vi "AlliGator All ROIs Average Lifetimes.vi"(8 "error in (no error)":errorcluster, 10 "Lifetime Graph":refnum<vi>, 11 "AlliGator Internal Variables DVR":refnum<data-value>) -> (0 "error out":errorcluster, 1 "Message":string, 3 "AlliGator Internal Variables DVR":refnum<data-value>)   [LabVIEW 2021, in "AlliGator Decay Processing.lvlib"]
doc: "Computes an approximate average lifetime for all ROI decays, based on the integral under the curve and IRF information."
uses:
  AlliGator Decay Processing.lvlib
  Internal Variables/AlliGator Internal Variables v2.ctl
  <vilib>/vision/Image Controls.llb/IMAQ Image.ctl
  Internal Variables/AlliGator Gate Image Set.ctl
  Files/AlliGator FLI Dataset Type.ctl
  Files/AlliGator Data Series Type.ctl
  Dual-Channel Datasets/AlliGator Dataset Channel.ctl
  Settings/AlliGator Gate Arithmetic.ctl
  Source Image/AlliGator Displayed Image.ctl
  Image/Named ROI Description.ctl
  Phasor Graph/AlliGator Decay Metadata v3.ctl
  Decay Preprocessing/AlliGator Decay Background Subtraction Info.ctl
  Decay Preprocessing/AlliGator Baseline Subtraction Method.ctl
  Graphs/XY Graph/XY Graph Plot Shift Parameters.ctl
  Graphs/XY Graph/XY Graph Plot Shift Method.ctl
  Decay Preprocessing/AlliGator Decay Extrapolation Parameters.ctl
  Phasor/Calibration Phasor (m, phi).ctl
  Phasor/Phasor Reference Series.ctl
  Phasor/Phasor Calibration Map v2.ctl
  Phasor/Phasor (g, s).ctl
  Phasor Graph/AlliGator Raw Phasor Plot Data v5.ctl
  Phasor/Phasor Standard Deviation Options.ctl
  Phasor Plot/AlliGator Phasor Multi-Harmonic Data.ctl
  Phasor/Phasor Harmonic Data.ctl
  Decay Fit Parameter Map/AlliGator Decay Fit Options & Parameters v4.ctl
  Fits/Decay Convolution/Decay Model.ctl
  Fits/Residual Type.ctl
  Fits/Non-linear Fitting Method v2.ctl
  Fits/Fit Calculation Method.ctl
  Fits/Non-linear Fitting Algorithm.ctl
  Decay Preprocessing/AlliGator Decay Preprocessing Parameters.ctl
  Fits/IRF(X)PSED/Decay Fit Parameters & Derived Quantities List v2.ctl
  Fits/IRF(X)PSED/Decay Fit Result Constraint.ctl
  Decay Fit Parameter Map/AlliGator Parameter Maps Data.ctl
  Globals, Variables, Constants/AlliGator Variables List.ctl
  Settings/AlliGator Average Lifetime Options.ctl
  Settings/AlliGator Settings List.ctl
  Rich Text Box/Text Format List.ctl
  Variant/Variant to Data/Variant to U16.vi
  Variant/Variant to Data/Variant to Boolean.vi
  Globals, Variables, Constants/AlliGator Abort.vi
  <vilib>/Utility/error.llb/Error Cluster From Error Code.vi
  <vilib>/ErrorRing/Error Ring.xnode
  Fits/IRF(X)PSED/MLE Baseline Offset Type.ctl
  Decay Fit/AlliGator Decay Fit Parameter Constraints 2.ctl
  Fits/IRF(X)PSED/Decay Fit Parameters In List.ctl
  Globals, Variables, Constants/AlliGator Globals, Variables & Constants.lvlib
  Image/Image.lvlib
  Source Image/AlliGator Source Image.lvlib
  Strings/Strings.lvlib
  Time/Time.lvlib
  Graphs/XY Graph/XY Graph Add-Ons.lvlib
  Settings/AlliGator Settings.lvlib
  Decay Preprocessing/AlliGator Decay Preprocessing.lvlib
  Variant/Variant to Data/Variant to Data.lvlib
  Notebook/Notebook.lvlib
  Fits/Fits.lvlib
  IRF/AlliGator IRF.lvlib
  Utilities/Utilities.lvlib
  GUI/GUI.lvlib
  Decay Fit Parameter Map/AlliGator Decay Fit Parameter Map.lvlib
  Decay Fit/AlliGator Decay Fit.lvlib
  Fits/IRF(X)PSED/Fit Weights Type v2.ctl
  Fits/IRF(X)PSED/Decay Fit Options v4.ctl
  Phasor/Phasor.lvlib
  Files/AlliGator Files.lvlib
  Internal Variables/AlliGator Internal Variables.lvlib
  Phasor Graph/AlliGator Phasor Graph.lvlib
  Phasor Plot/AlliGator Phasor Plot.lvlib
  Dual-Channel Datasets/AlliGator Dual-Channel Datasets.lvlib
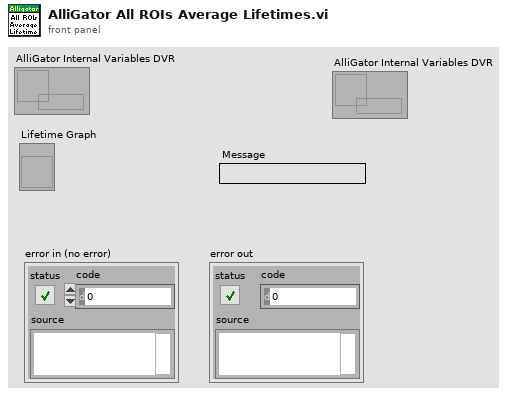
[diagram p1: front panel]
types:
  T1 = typedef "AlliGator Globals, Variables & Constants.lvlib/AlliGator Variables List.ctl" = enum16{"---- GUI ----", "GUI:Initialization Status", "GUI:State Indicators Refnum", "GUI:Original AlliGator Menu Items", "GUI:Current Action Loop State", "GUI:Script in progress", "GUI:Playback", "GUI:Loop Playback", "GUI:Search ROI Used", "GUI:Search ROI", "Decay Graph Max Legend Size", "Intensity Graph Max Legend Size", "Decay Statistics Graph Max Legend Size", "Phasor Graph Max Legend Size", "Phasor Ratio Graph Max Legend Size", "Lifetime Graph Max Legend Size", "---- Files ----", "Files:Export Dataset Frames as Individual Files", "Files:Show Batch Export Help Balloons", "Files:Frames in Dataset", "Files:ptu File Frame Start Indices", "Files:Current Frame in Dataset", "Files:Current Frame Timestamp", "Files:Dataset Loaded", "Files:Dataset Metadata", "Files:Dataset Channel", "Files:Dataset Data Description", "Files:Background Dataset Metadata", "Files:Background Dataset Channel", "Files:Background Dataset Data Description", "Files:Background File Subtraction", "Files:Background File Path", "Files:Background File Pile-up Correction", "Files:Background File Pixel Well Capacity", "Files:Background File Scaling Factor", "Files:Current Dataset Load Settings", "Files:Dataset Path", "Files:ICCD-specific Information", "Files:Macrotime Gate Separation", "------ Python Plugins ------", "Python Plugins:Information", "Python Plugins:Python Session", "Python Plugins:Valid Python Session?", "---- Source Image ----", "Source Image:ROIs", "Source Image:Current ROI", "Source Image:ROI Event Refnum", "X_Source Image:Display Range", "X_Source Image:Palette Information", "X_Source Image:Type of Displayed Image", "X_Time Gate Slider", "Source Image:Palette List", "Source Image:Scale", "Source Image:ROI Overlay Color", "Source Image:Overlay to Erase", "Source Image:Is Displayed Image Accumulated", "Source Image:White Light Image Modified", "Source Image:Mask Image Modified", "---- Image Profile Window ----", "Image Profile:Window Event Refnum", "Image Profile:IntensityType", "Image Profile:Intensity Average Type", "Image Profile:Intensity-weighted SDV", "Image Profile:Box Profile Type", "Image Profile:Window Open", "Image Profile:Plotted Fit Parameter", "------ Phasor Graph -------", "Phasor Graph:Show Line", "---- Phasor Plot ---", "Phasor Plot:Parameters Changed", "Phasor Plot:FLI Dataset Modified since last Calculation", "Phasor Harmonics Data", "Selected Phasor Harmonics", "Phasor Harmonic Manager Event Refnum", "Phasor Plot:ROIs", "Phasor Plot:Current ROI", "Phasor Plot:ROI Event Refnum", "Phasor Plot:Image Reference Points", "Phasor Plot:Computed", "Phasor Plot:Palette Information", "Phasor Plot:Palette List", "Phasor Plot:Phasor Ratio Palette Information", "Phasor Plot:Phasor Ratio Palette List", "Phasor Plot:Image Scale", "Phasor Plot:Image Overlay to Erase", "Phasor Plot:Image Elements to Update", "Phasor Plot:Current Calculation Parameters", "Phasor Plot:Current Calibration Options", "Phasor Plot:Reset Cumulated Phasor Plot", "Phasor Plot:Reference 1", "Phasor Plot:Lifetime Reference 1", "Phasor Plot:Reference 1 Frequency", "Phasor Plot:Reference 2", "Phasor Plot:Lifetime Reference 2", "Phasor Plot:Reference 2 Frequency", "---- Decay Analysis ----", "Number of Selected Decays to Fit", "LS Fit Results", "LAR Fit Results", "BS Fit Results", "Last Decay Max - Min", "Best Fit Parameters", "Best Fit Parameter Names", "Actual Size X", "Actual Size Y", "Binning X", "Binning Y", "Actual # Gates", "Dataset Number", "Gates to...", "Gates Skipped", "Gates to keep", "Gate Step", "Gate Separation", "Reversed Gates", "Pile-up Correction", "Pixel Well Capacity", "Background Subtracted", "Background Subtraction Method", "Background Definition Range", "Background File (deprecated)", "Number of Dataset Accumulated", "Array of Accumulated Dataset Paths", "Do Averaged Datasets", "Destination File Path", "Process Plot Target", "Use 1/D as Phasor Frequency", "---- Decay Fit Parameter Map -----", "Decay Fit Parameter Map:Palette Information", "Decay Fit Parameter Map:Palette List", "Decay Fit Parameter Map:X Resolution", "Decay Fit Parameter Map:Y Resolution", "Decay Fit Parameter Map:Use Decay Fit Result Constraints", "Decay Fit Parameter Map:Decay Fit Result Constraints", "Decay Fit Parameter Map:Decay Fit Result Constraints Applied", "---- Parameter Map ----", "Parameter Map:Palette Information", "Parameter Map:Palette List", "------- Local Decay Window ---------", "Local Decay Graph Window:Event Refnum", "Local Decay Graph Window:Use normalized IRF for convolution", "----- Miscellaneous ----", "Misc:Skippable Dialog Windows Status"}
  T2 = typedef "AlliGator Settings.lvlib/AlliGator Average Lifetime Options.ctl" = cluster{"Use Local IRF ":bool, "Use IRF Offset":bool, "Use Fixed Offset":bool, "Fixed Offset":dbl[unit], "Baseline %":dbl}
  T3 = typedef "AlliGator Settings.lvlib/AlliGator Settings List.ctl" = enum16{"GUI:Visible Settings Tab", "GUI:Last Run Version", "Source Image:Use Image Histogram for Contrast", "Source Image:Low Count Pixels Rejection Options", "Source Image:High Count Pixels Rejection Options", "Source Image:Use Image Brightness", "Source Image:Blend Overlay with Image Background", "Source Image:Use Fixed ROI Diameter", "Source Image:ROI Diameter", "Source Image:ROI Center Color", "Source Image:Peak Threshold", "Source Image:Intensity Threshold", "Source Image:Image Binning Options", "Source Image:Image Smoothing Options", "Source Image:Image Histogram Active", "Source Image:Invert Binary Mask", "Source Image:Hot Pixel Removal", "Source Image:Overlay Analyzed ROI Center", "Source Image:Auto-Adjust Contrast", "Source Image:Histogram Lower Percentile", "Source Image:Histogram Upper Percentile", "Source Image:Save Source Image", "Source Image:Scale Bar Options", "Source Image:Image Resolution (Pixel Size)", "Source Image:Flatfield Correction", "Source Image:Show Dead Left Columns Correction", "Source Image:Dead Left Columns Correction", "Source Image:Image Pre-Processing Operations Order", "Source Image:Overlay ROI Median", "Source Image:Median Overlay Color", "Data Information:Gate Width", "Data Information:Nanotime Gate Separation", "Data Information:Macrotime Gate Separation", "Data Information:Gate Step", "Data Information:# Gates", "Data Information:Gate Image Exposure", "Data Information:Gate Image Integration", "Data Information:Gates to Skip", "Data Information:Gates to Keep", "Data Information:Define Gates to", "Data Information:Channel Name", "Data Information:Available Channel Names", "Data Information:Channel Arithmetic", "Data Information:Background File Subtraction", "Data Information:Background File", "Data Information:Background Scaling Factor", "Data Information:Background Pile-up Correction", "Data Information:Background Pixel Well Capacity", "Data Information:Laser Period", "Data Information:SYNC Period", "Data Information:Pile-up Correction", "Data Information:Pixel Well Capacity", "Data Information:Dataset Scaling Factor", "Fluorescence Decay_Decay Pre-Processing:Reverse Gates", "Fluorescence Decay_Decay Pre-Processing:Verbose Decay Pre-Processing", "Fluorescence Decay_Decay Pre-Processing:Use Decay Pre-Processing", "Fluorescence Decay_Decay Pre-Processing:Background Subtraction", "Fluorescence Decay_Decay Pre-Processing:Background Definition Range", "Fluorescence Decay_Decay Pre-Processing:Baseline Subtraction Method", "Fluorescence Decay_Decay Pre-Processing:Decay Pre-Processing Operations Order", "Fluorescence Decay_Decay Pre-Processing:Smoothing Parameter", "Fluorescence Decay_Decay Pre-Processing:Shift Decay", "Fluorescence Decay_Decay Pre-Processing:Decay Shift Parameters", "Fluorescence Decay_Decay Pre-Processing:Fold Decay", "Fluorescence Decay_Decay Pre-Processing:# Folds", "Fluorescence Decay_Decay Pre-Processing:1-Normalize Decay", "Fluorescence Decay_Decay Pre-Processing:[0-1]-Normalize Decay", "Fluorescence Decay_Decay Pre-Processing:Smoothen Decay", "Fluorescence Decay_Decay Pre-Processing:Extrapolate Decay", "Fluorescence Decay_Decay Pre-Processing:Use Periodicity", "Fluorescence Decay_Decay Pre-Processing:Use Cursors", "Fluorescence Decay_Decay Pre-Processing:Tail Fraction", "Fluorescence Decay_Decay Pre-Processing:Head Fraction", "Fluorescence Decay_Decay Pre-Processing:Additional Points", "Fluorescence Decay_Decay Pre-Processing:Straighten Decay", "Fluorescence Decay_Decay Pre-Processing:Constant Background", "Fluorescence Decay_Decay Pre-Processing:Pixel-Normalize Decay", "Fluorescence Decay_Advanced Analysis:Extract IRF instead of Decay", "Fluorescence Decay_Advanced Analysis:IRF Extraction Options", "Fluorescence Decay_Advanced Analysis:IRF Optimization Options", "Fluorescence Decay_Advanced Analysis:Square Pulse Options", "Fluorescence Decay_Advanced Analysis:IRF Order", "Fluorescence Decay_Advanced Analysis:IRF Time Constants", "Fluorescence Decay_Advanced Analysis:Wavelet Analysis Options", "Fluorescence Decay_Advanced Analysis:Average Lifetime Options", "Fluorescence Decay_Fit Options:Fit Options", "Fluorescence Decay_Fit Options:Use Legacy Fitting Approach", "Fluorescence Decay_Fit Options:Use Data Information Laser Period", "Fluorescence Decay_Fit Parameters:Displayed Fit Parameters", "Fluorescence Decay_Fit Parameters:Fit Parameter Constraints", "Fluorescence Decay_Fit Parameters:Export Tabulated Results", "Fluorescence Decay_Fit Parameters:MLE Baseline Offset Type", "Fluorescence Decay_Fit Parameters:MLE Baseline Offset", "Fluorescence Decay_Fit Parameters:Guess Parameter Names", "Fluorescence Decay_Fit Parameters:Guess Parameter Values", "Fluorescence Decay_Fit Parameters:Guess Parameters Options", "Fluorescence Decay_Fit Parameters:Optimal Offset Selection Criterion", "Fluorescence Decay_Styles:Show Last Decay Only", "Fluorescence Decay_Styles:Decay Graph Color Array", "Fluorescence Decay:Decay Graph Active", "Fluorescence Decay Statistics:Min Peak Value", "Fluorescence Decay Statistics:Reject Low Decay Peak Pixels", "Fluorescence Decay Statistics:Reject High Decay Peak Pixels", "Fluorescence Decay Statistics:Max Peak Value", "Time Traces:Use File Timestamp", "Time Traces:Time Step", "Time Traces:Use Intensity Correction File", "Time Traces:Intensity Correction File", "Phasor Plot:Phasor Plot Smoothing Options", "Phasor Plot:Phasor Plot Size", "Phasor Plot:Phasor Plot Graphics Options", "Phasor Plot:Cumulative Phasor Plot", "Phasor Plot:Use Phasor Brightness", "Phasor Plot:Blend Overlay with Phasor Background", "Phasor Plot:Save Phasor Plot", "Phasor Plot:Show References", "Phasor Plot:Phasor Ratio Decay Range", "Phasor Plot:Exponential Fading", "Phasor Plot:Phasor Ratio Reference Colors", "Phasor Plot:Reference Radius", "Phasor Plot:Show Color Map Vertices", "Phasor Plot:Phasor Plot Active", "Phasor Plot:Phasor Ratio Color Map Type", "Phasor Plot:Phasor Ratio Color Map", "Phasor Plot:Phasor Ratio Display Range", "Phasor Plot:Selected Image ROI(s)", "Phasor Plot:All Image ROIs", "Phasor Plot:Selected Phasor Plot ROI(s)", "Phasor Plot:All Phasor Plot ROIs", "Phasor Plot:Phasor Ratio Color-Coded Quantity", "Phasor Plot:Store Phasor Harmonics", "Phasor Plot:Draw Reference Segment", "Phasor Plot:User-Defined Quantity", "Phasor Plot:Color Scale High Color", "Phasor Plot:Color Scale Low Color", "Phasor Plot:Intensity-weighted Phasor Plot", "Phasor Graph:Phasor Frequency", "Phasor Graph:Phasor Ratio Type", "Phasor Graph:Pixel-level Phasor Computation", "Phasor Graph:Save Phasor Graph", "Phasor Graph:Phasor Graph Active", "Phasor Graph:Phasor SDV Options", "Phasor Graph:Intensity-weighted Phasor Graph", "Phasor Graph:Define Shortest Lifetime as", "Phasor Calibration:Use Backup Calibration if needed", "Phasor Calibration:Backup Calibration Type", "Phasor Calibration:Calibration Type", "Phasor Calibration:Calibration Lifetime", "Phasor Calibration:Calibration Map Algorithm", "Single-Exponential Phasor Locus (SEPL):Gate Parameters", "Single-Exponential Phasor Locus (SEPL):User-defined Gate", "Single-Exponential Phasor Locus (SEPL):User-defined IRF", "Single-Exponential Phasor Locus (SEPL):Phasor Parameters", "Single-Exponential Phasor Locus (SEPL):Decay & IRF Parameters", "Single-Exponential Phasor Locus (SEPL):Display Parameters", "Lifetime Analysis:Decay Analysis Parameters", "Lifetime Analysis:Lifetime Map Active", "Plugins:Python Settings", "Miscellaneous:Verbose Mode", "Miscellaneous:Beep after Script", "Miscellaneous:Saved Image File Format", "Miscellaneous:Exported Gate Image Settings", "Miscellaneous:Include Loading in Timing", "Miscellaneous:Verbose Settings Mode", "Miscellaneous:Histogram Options", "Miscellaneous:Beep on Error", "Miscellaneous:# Logical Processors Used", "Miscellaneous:ROI Description Max Characters", "Miscellaneous:Verbose Error Mode", "Miscellaneous:Transparent Mask Color"}
  T4 = typedef "IMAQ Image.ctl" = refnum<image>
  T5 = typedef "Image.lvlib/Named ROI Description.ctl" = cluster{"ROI Descriptor":T6, "ROI Name":string, "Overlay Color":u32}
  T6 = typedef "ROI Descriptor" = cluster{"Global Rectangle":i32[], "Contours":cluster{"ID":enum32{"External", "Internal"}, "Type":u32, "Coordinates":i32[]}[]}
  T7 = typedef "Notebook.lvlib/Text Format List.ctl" = enum16{"Message", "Result", "Error", "Setting", "Verbose", "Warning"}
  T8 = typedef "AlliGator Decay Fit Parameter Map.lvlib/AlliGator Decay Fit Options & Parameters v4.ctl" = cluster{"SYNC Period":dbl[unit], "Fit Options":T9, "Fit Parameter Constraints":T16[], "MLE Baseline Offset":dbl, "MLE Baseline Offset Type":T18}
  T9 = typedef "Fits.lvlib/Decay Fit Options v4.ctl" = cluster{"Show Fit Residuals":bool, "Fit Model":T10, "Residual Type":T11, "Max Decay Percentile":dbl, "Min Decay Percentile":dbl, "Show Full Decay":bool, "Weights":T12, "Fitting Method":T13, "Compute Parameter Uncertainties":bool, "Periodic Boundaries":bool, "Model Calculation":T14, "Period":dbl[unit], "Termination Criteria":cluster{"Max Iterations":i32, "Max Function Calls":i32, "Max Time":dbl[unit], "Function Tolerance":dbl, "Parameter Tolerance":dbl, "Gradient Tolerance":dbl, "Min Lambda":dbl, "Max Lambda":dbl, "Initial Tick Count":u32}, "Offset Resolution":dbl[unit], "Use Local IRF":bool, "Fitting Algorithm":T15, "Show Confidence Interval ":bool, "Confidence Level":dbl}
  T10 = typedef "Fits.lvlib/Decay Model.ctl" = enum16{"1-Exponential", "2-Exponentials"}
  T11 = typedef "Fits.lvlib/Residual Type.ctl" = enum16{"Standard", "Normalized", "Reduced"}
  T12 = typedef "Fits.lvlib/Fit Weights Type v2.ctl" = enum16{"Unweighted", "1/Variance (Neyman)", "1/Variance (Pearson)", "Best of All"}
  T13 = typedef "Fits.lvlib/Non-linear Fitting Method v2.ctl" = enum16{"Least Square", "Least Absolute Residual", "Bisquare", "MLE", "-", "Best of All"}
  T14 = typedef "Fits.lvlib/Fit Calculation Method.ctl" = enum16{"Simulation", "Convolution", "Integration"}
  T15 = typedef "Fits.lvlib/Non-linear Fitting Algorithm.ctl" = enum16{"Levenberg-Marquardt", "Trust-Region Dogleg"}
  T16 = typedef "AlliGator Decay Fit.lvlib/AlliGator Decay Fit Parameter Constraints 2.ctl" = cluster{"Fit Parameter":T17, "Min Value":dbl, "Max Value":dbl, "Global":bool, "Used":bool}
  T17 = typedef "Fits.lvlib/Decay Fit Parameters In List.ctl" = enum16{"Offset", "Baseline", "A_1", "tau_1", "A_2", "tau_2"}
  T18 = typedef "Fits.lvlib/MLE Baseline Offset Type.ctl" = enum32{"Absolute", "Percentage"}
  T19 = typedef "AlliGator Internal Variables.lvlib/AlliGator Internal Variables v2.ctl" = cluster{"----------------------------- Images -----------------------------":u8, "Displayed Image":T4, "White Light Image":T4, "Mask Image":T4, "ROI Mask Image":T4, "Current Dataset Images 1":T20, "Background Dataset Images 1":T20, "Current Dataset Images 2":T20, "Background Dataset Images 2":T20, "Current Dataset Arithmetic Images":T20, "Accumulated Dataset Images 1":T20, "Accumulated Dataset Images 2":T20, "Accumulated Dataset Arithmetic Images":T20, "----------------------------- File Paths -----------------------------":u8, "Phasor Plot Image":T4, "Decay Fit Parameter Map Image":T4, "Parameter Map Image":T4, "Single Data Point Path":path, "White Light Image Path":path, "Mask Image Path":path, "Time-Series Folder":path, "[Time-Series Paths]":path[], "----------------------------- FLI Dataset -----------------------------":u8, "Current Dataset":i32, "Single Dataset Type":T21, "Current Folder":string, "AlliGator Data Series Type":T22, "# Datasets":i32, "Dual-Channel Dataset":bool, "Selected Channel Name":string, "Dataset Channel":T23, "Channel Arithmetic":T24, "Dual-Channel Background Dataset":bool, "Background Channel":T23, "Dual-Channel Accumulated Dataset":bool, "Start Time":dbl, "[Time-Series Timestamps]":dbl[], "[Intensity Corrections]":dbl[], "Time Series Script":bool, "Type of Displayed Image":T25, "Gate Image Slide":u16, "# Gates":i32, "ROIs":T5[], "----------------------------- Decays -----------------------------":u8, "ROI Decay":cluster{"t Array":dbl[], "I Array":dbl[]}, "Valid Decay":bool, "Decay  Metadata":T26, "Reference Decay Plot Name":string, "Reference Decay":cluster{"t Array":dbl[], "I Array":dbl[]}, "Decay Shift Plot":cluster{"Time Stamps":dbl[], "Decay Shifts":dbl[]}, "[Decays Max Values]":sgl[], "[Decays Min Values]":sgl[], "----------------------------- Calibration -----------------------------":u8, "Calibration Phasor":T32, "Calibration Phasor Series":T33, "Phasor Calibration Map":T34, "Calibration Map MD5 Digest":string, "----------------------------- Phasor Graph -----------------------------":u8, "Last Raw Phasor":T35, "Last Calibrated Phasor":T35, "Last Calibrated Phasor SDV":T35, "Phasor Graph:Phasor Plot":cluster{"g Array":dbl[], "s Array":dbl[]}, "Phasor Graph:Phasor SDV Plot":cluster{"g Array":dbl[], "s Array":dbl[]}, "[Phasor Graph:Raw Phasor Plots]":T36[], "Phasor Plot locked to Ref 1":i32, "[Phasor Plot(s) locked to Ref 1]":i32[], "[Phasor Plot(s) locked to Ref 2]":i32[], "[Pixel Phasors]":T35[], "----------------------------- Phasor Plot -----------------------------":u8, "[[Sum Image]]":dbl[][], "[[CSG Phasors]]":csg[][], "[[Valid Pixel?]]":bool[][], "[[Phasor Ratios]]":dbl[][], "[[Average Lifetimes]]":dbl[][], "Amplitude Weighted Average Lifetime":bool, "I/m/phi Dataset":cluster{"I/m/phi Dataset?":bool, "Base Frequency":dbl[unit], "Harmonic Orders":u8[]}, "Multi Phasor Plot Data":T38, "----------------------------- Decay Fit Parameter Map -----------------------------":u8, "Decay Fit Options & Parameters":T8, "Fit Options: Decay Preprocessing Parameters":T40, "Fit Options: Reference Decay":cluster{"t Array":dbl[], "I Array":dbl[]}, "Is Full Image Parameters Map":bool, "Is Single-Pixels Parameters Map":bool, "NLSF Parameters Map X Resolution":i32, "NLSF Parameters Map Y Resolution":i32, "[Single Decay Fit Parameters]":dbl[], "Fit Model":T10, "[[Multiple Decays Fit Parameters]]":dbl[][], "[[Multiple Decays Fit Parameter SDVs]]":dbl[][], "[[IRFs]]":dbl[][], "[ROI Descriptors]":T6[], "IRF Array Time Axis":dbl[], "Decay Array Time Axis":dbl[], "[Decay Fit Parameter Names]":T41[], "[Decay Sum]":dbl[], "Array of Decay Fit Result Constraints":T42[], "Selected ROIs Array":bool[], "----------------------------- Parameter Maps -----------------------------":u8, "[Map Set Names]":string[], "[Parameter Maps]":T43[], "[[User-defined Quantities]]":dbl[][], "User-defined Quantity":string}
  T20 = typedef "AlliGator Internal Variables.lvlib/AlliGator Gate Image Set.ctl" = cluster{"SGL Image Max":T4, "SGL Image Sum":T4, "SGL Gate Images":T4[], "SGL Image Min":T4}
  T21 = typedef "AlliGator Files.lvlib/AlliGator FLI Dataset Type.ctl" = enum16{"HDF5 FLI Dataset", "Gate Image Folder", ".sdt FLI Dataset (Becker & Hickl)", ".ptu FLI Dataset (PicoQuant)", "SS1 FLI Dataset", "SS2 FLI Dataset", "I/m/phi Dataset", ".bin FLI Dataset (PicoQuant Binned)", ".bin FLI Dataset (Piccolo Binned)", ".mat FLI Dataset"}
  T22 = typedef "AlliGator Files.lvlib/AlliGator Data Series Type.ctl" = enum16{"Not a Supported Series", "Gate Images Folder Series", "SwissSPAD 2 Dataset Series", "B&H FLI Dataset Series", "PicoQuant PTU FLI Dataset Series", "PicoQuant BIN FLI Dataset Series", "Piccolo hist BIN FLI Dataset Series", "HDF5 FLI Dataset Series"}
  T23 = typedef "AlliGator Dual-Channel Datasets.lvlib/AlliGator Dataset Channel.ctl" = enum16{"G2", "INT"}
  T24 = typedef "AlliGator Settings.lvlib/AlliGator Gate Arithmetic.ctl" = enum16{"None", "INT-G2", "G2/INT*<INT>", "(1 - G2/INT)*<INT>"}
  T25 = typedef "AlliGator Source Image.lvlib/AlliGator Displayed Image.ctl" = enum16{"Single Gate", "Sum of All Gates", "Max of All Gates", "Min of All Gates", "-", "White Ligth Image", "Mask Image"}
  T26 = typedef "AlliGator Phasor Graph.lvlib/AlliGator Decay Metadata v3.ctl" = cluster{"ROI Descriptor":T6, "ROI Center":cluster{"X":i32, "Y":i32}, "Decay Background Subtraction Info":T27, "Decay Reverted":bool, "Decay Smoothened":bool, "Decay Straightened":bool, "Fitted Tau (Decay Straightening)":dbl, "Decay Shift Parameters":T29, "Decay Shifted":bool, "Decay Extrapolated":bool, "Decay Extrapolation Parameters":T31, "Decay Normalized":bool, "Fold Decay":bool, "# Folds":u32}
  T27 = typedef "AlliGator Decay Preprocessing.lvlib/AlliGator Decay Background Subtraction Info.ctl" = cluster{"Laser Period":dbl[unit], "Gate Duration":dbl[unit], "Baseline Subtraction Method":T28, "Background Definition Range":cluster{"Min Gate":dbl[unit], "Max Gate":dbl[unit]}, "Total Intensity w/o Bkgd Subtraction":dbl, "Bkgd-subtracted Intensity (exp)":dbl, "# Data Points":i32, "Background/Gate":dbl, "Fitted Lifetime":dbl[unit], "Bkgd-subtracted Intensity (theo)":dbl}
  T28 = typedef "AlliGator Decay Preprocessing.lvlib/AlliGator Baseline Subtraction Method.ctl" = enum16{"Mean", "Min", "Square Gated Single-Exponential", "File", "Constant"}
  T29 = typedef "XY Graph Add-Ons.lvlib/XY Graph Plot Shift Parameters.ctl" = cluster{"Type":T30, "Shift":dbl[unit], "Threshold":dbl, "Rotate":bool}
  T30 = typedef "XY Graph Add-Ons.lvlib/XY Graph Plot Shift Method.ctl" = enum16{"Default", "CFD", "Threshold", "Cross-Correlation"}
  T31 = typedef "AlliGator Decay Preprocessing.lvlib/AlliGator Decay Extrapolation Parameters.ctl" = cluster{"Additional Points":u32, "Head Fraction":dbl, "Fitted Tau":dbl, "Use Periodicity":bool, "Use Cursors":bool, "Tail Fraction":dbl}
  T32 = typedef "Phasor.lvlib/Calibration Phasor (m, phi).ctl" = cluster{"m":dbl, "phi":dbl, "Phasor Frequency":dbl[unit], "Reference Lifetime":dbl[unit]}
  T33 = typedef "Phasor.lvlib/Phasor Reference Series.ctl" = cluster{"m Array":dbl[], "phi Array":dbl[], "Phasor Frequency":dbl[unit], "Calibration Lifetime":dbl[unit]}
  T34 = typedef "Phasor.lvlib/Phasor Calibration Map v2.ctl" = cluster{"Phasor Frequency":dbl[unit], "Calibration Lifetime":dbl[unit], "ROI Centers":cluster{"X":i32, "Y":i32}[], "ROI Descriptors":T6[], "Map Resolution X":i32, "Map Resolution Y":i32, "z Array":cdb[]}
  T35 = typedef "Phasor.lvlib/Phasor (g, s).ctl" = cluster{"g":dbl, "s":dbl}
  T36 = typedef "AlliGator Phasor Graph.lvlib/AlliGator Raw Phasor Plot Data v5.ctl" = cluster{"Phasor Plot Name":string, "Raw Phasor Plot":T35[], "Phasor Frequency":dbl[unit], "[Decay Metadata]":T26[], "Raw Phasor Plot SDV":T35[], "Phasor SDV Options":T37, "[Calibration Phasor]":T32[], "Intensity Array":dbl[]}
  T37 = typedef "Phasor.lvlib/Phasor Standard Deviation Options.ctl" = cluster{"Compute Estimated SDV":bool, "# Replicas":u32, "Use Estimated Average Phasor":bool}
  T38 = typedef "AlliGator Phasor Plot.lvlib/AlliGator Phasor Multi-Harmonic Data.ctl" = cluster{"Base Frequency":dbl[unit], "# Harmonics":u8, "Harmonic Orders":u8[], "Phasor Plot Settings Checksum":u64, "Phasor Harmonic Data Array":T39[]}
  T39 = typedef "Phasor.lvlib/Phasor Harmonic Data.ctl" = cluster{"Phasor Harmonic Name":string, "Phasor Plot Settings Checksum":u64, "Phasor Frequency":dbl[unit], "Base Frequency":dbl[unit], "Harmonic Order":u8, "Phasor Plot Parameters":string, "Phasor Array [[CSG]]":csg[][], "Dataset File Path":path}
  T40 = typedef "AlliGator Decay Preprocessing.lvlib/AlliGator Decay Preprocessing Parameters.ctl" = cluster{"Background Subtraction":bool, "Straighten Decay":bool, "Reverse Gates":bool, "1-Normalized Decay":bool, "Smoothen Decay":bool, "Smoothing Parameter":dbl, "Shift Decay":bool, "Decay Shift Parameters":T29, "Extrapolate Decay":bool, "Additional Points":u32, "Head Fraction":dbl, "Pixel-Normalize Decay":bool, "Use Periodicity":bool, "Use Cursors":bool, "Tail Fraction":dbl, "Use Decay Pre-Processing":bool, "Fold Decay":bool, "# Folds":u32, "[0-1]-Normalized Decay":bool}
  T41 = typedef "Fits.lvlib/Decay Fit Parameters & Derived Quantities List v2.ctl" = enum16{"Offset", "Baseline", "A_1", "tau_1", "A_2", "tau_2", "<tau>_a", "f1_a", "f2_a", "<tau>_i", "f1_i", "f2_i", "-", "R^2", "Chi^2"}
  T42 = typedef "Fits.lvlib/Decay Fit Result Constraint.ctl" = cluster{"Fit Parameter":enum16{"Offset", "Baseline", "A_1", "tau_1", "A_2", "tau_2", "<tau>_a", "f1_a", "f2_a", "<tau>_i", "f1_i", "f2_i", "-", "R^2", "Chi^2", "Max Relative Residual", "<Residual ACF>", "Residual ACF SDV", "tau_2/tau_1"}, "Min Value":dbl, "Max Value":dbl, "Use Constraint":bool}
  T43 = typedef "AlliGator Decay Fit Parameter Map.lvlib/AlliGator Parameter Maps Data.ctl" = cluster{"Map Set Name":string, "[Parameter Names]":string[], "[[Parameters]]":dbl[][], "[[Parameter SDVs]]":dbl[][], "Decay Array Time Axis":dbl[], "[[IRFs]]":dbl[][], "IRF Array Time Axis":dbl[], "X Resolution":i32, "Y Resolution":i32, "Intensity Array":dbl[]}
  T44 = typedef "AlliGator Settings.lvlib/AlliGator Pixel Counts Constraints.ctl" = cluster{"High Count Pixels Rejection Options":T45, "Low Count Pixels Rejection Options":T46}
  T45 = typedef "AlliGator Settings.lvlib/AlliGator High Count Pixels Rejection Options.ctl" = cluster{"Background High Threshold Factor":dbl, "Fixed High Background Threshold":dbl, "Reject High Count Pixels":bool, "High Percentile":dbl}
  T46 = typedef "AlliGator Settings.lvlib/AlliGator Low Count Pixels Rejection Options.ctl" = cluster{"Background Low Threshold Factor":dbl, "Fixed Low Background Threshold":dbl, "Reject Low Count Pixels":bool, "Low Percentile":dbl}
  T47 = cluster{"Decay Peak Constraint":bool, "Min":dbl, "Max":dbl}
  T48 = typedef "Rich Text Box.lvlib/Text Formatting.ctl" = cluster{"Font":string, "Text Color":T49, "Background Color":T49, "Style":T50, "Font Size":dbl, "Alignment":T51}
  T49 = typedef "Rich Text Box.lvlib/Text Colors.ctl" = enum16{"Unchanged", "Black", "Blue", "Cyan", "Maroon", "Gray", "Violet", "Green", "Light Green", "Orange", "Yellow", "Magenta", "Red", "White"}
  T50 = typedef "Rich Text Box.lvlib/Text Style.ctl" = enum16{"Regular", "Bold", "Italic", "Underline", "Strikeout"}
  T51 = typedef "Rich Text Box.lvlib/Text Alignment.ctl" = enum16{"Left", "Right", "Center"}
  T52 = typedef "XY Graph Add-Ons.lvlib/XY Graph Refnum.ctl" = refnum<vi>
  T53 = cluster{"t Axis":dbl[], "ROI Intensity Array":dbl[]}
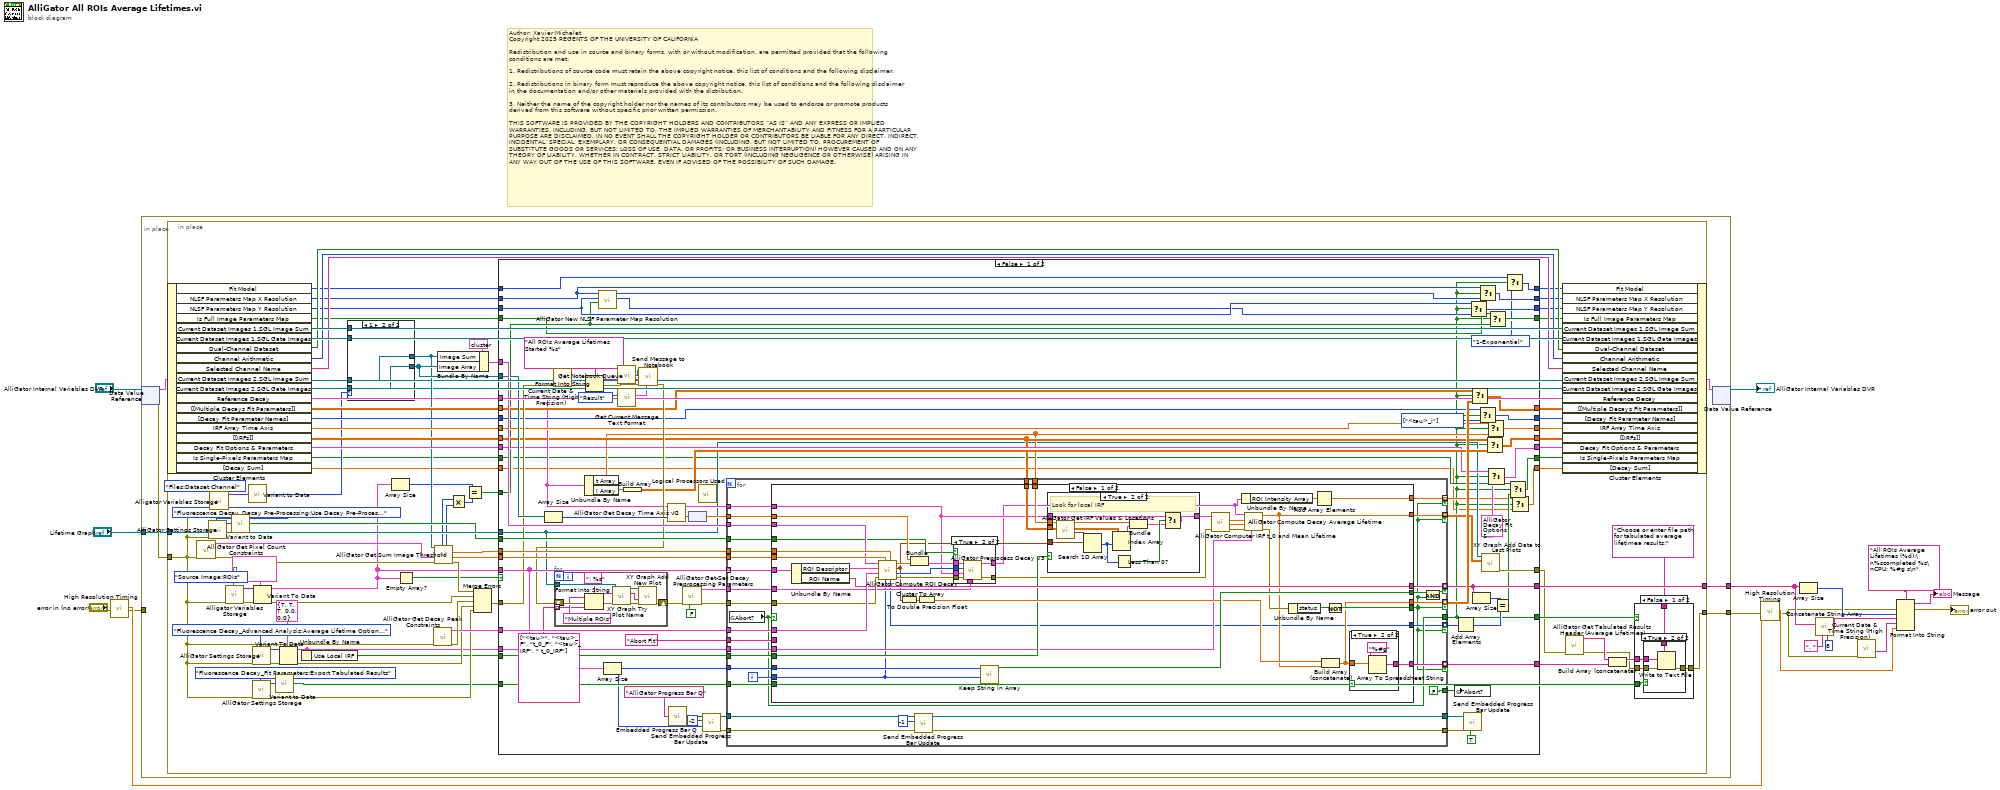
[diagram p0: block diagram]
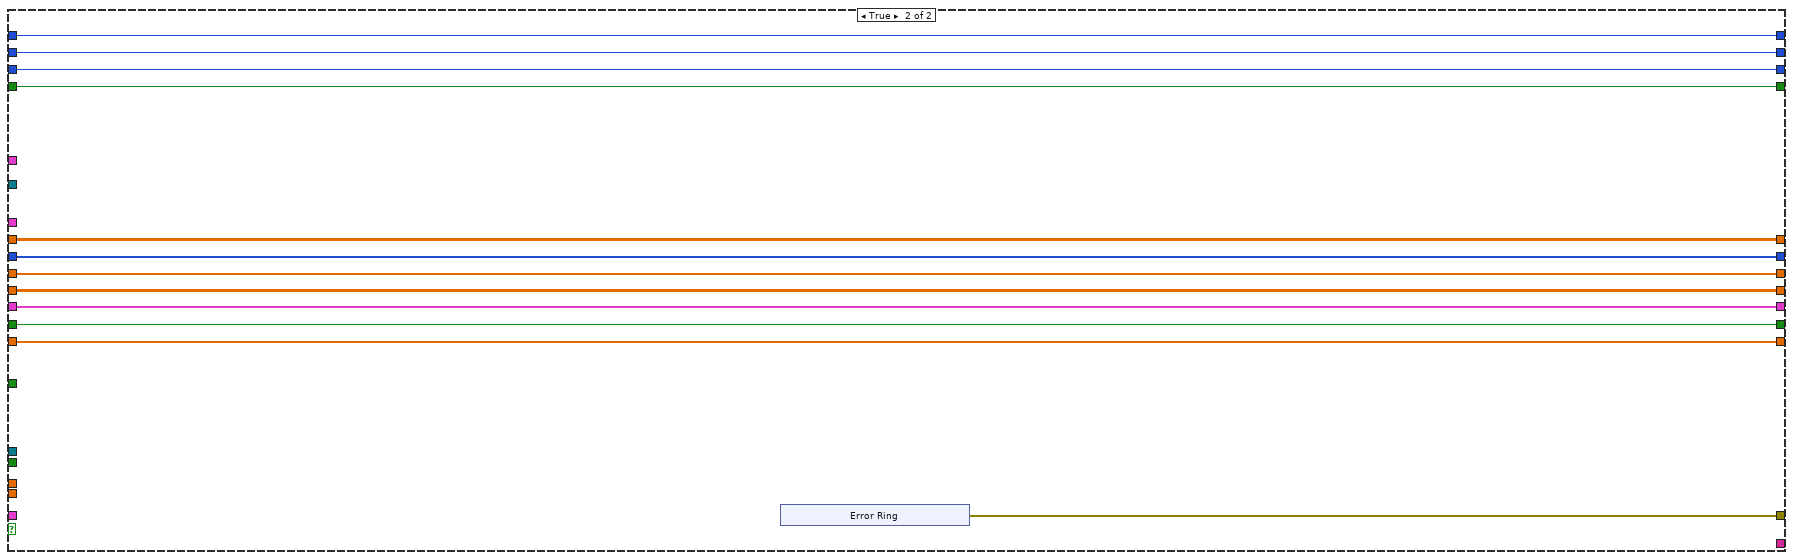
[diagram p7: hidden frame]
diagram:
  # "Author: Xavier Michalet\nCopyright 2025 REGENTS OF THE UNIVERSITY OF CALIFORNIA\n\nRedistribution and use in source and binary forms, with or without modification, are permitted provided that the following conditions are met:\n\n1. Redistributions of source code must retain the above copyright notice, this list of conditions and the following disclaimer.\n\n2. Redistributions in binary form must reproduce the above copyright notice, this list of conditions and the following disclaimer in the documentation and/or other materials provided with the distribution.\n\n3. Neither the name of the copyright holder nor the names of its contributors may be used to endorse or promote products derived from this software without specific prior written permission.\n\nTHIS SOFTWARE IS PROVIDED BY THE COPYRIGHT HOLDERS AND CONTRIBUTORS “AS IS” AND ANY EXPRESS OR IMPLIED WARRANTIES, INCLUDING, BUT NOT LIMITED TO, THE IMPLIED WARRANTIES OF MERCHANTABILITY AND FITNESS FOR A PARTICULAR PURPOSE ARE DISCLAIMED. IN NO EVENT SHALL THE COPYRIGHT HOLDER OR CONTRIBUTORS BE LIABLE FOR ANY DIRECT, INDIRECT, INCIDENTAL, SPECIAL, EXEMPLARY, OR CONSEQUENTIAL DAMAGES (INCLUDING, BUT NOT LIMITED TO, PROCUREMENT OF SUBSTITUTE GOODS OR SERVICES; LOSS OF USE, DATA, OR PROFITS; OR BUSINESS INTERRUPTION) HOWEVER CAUSED AND ON ANY THEORY OF LIABILITY, WHETHER IN CONTRACT, STRICT LIABILITY, OR TORT (INCLUDING NEGLIGENCE OR OTHERWISE) ARISING IN ANY WAY OUT OF THE USE OF THIS SOFTWARE, EVEN IF ADVISED OF THE POSSIBILITY OF SUCH DAMAGE."
  n1 = call "High Resolution Timing.vi"("Error In"="error in (no error)") -> ("elapsed (relative) seconds"=w12:dbl, "Error Out"=w7:errorcluster)  [unwired: 16 in, 1 out]
  n2 = in-place {
    in-place-border: [w22] -> w5
    in-place-border: [w21] -> w9
    in-place-border: w7 -> [_]
    in-place-border: "Lifetime Graph" -> [w19]
    n3 = in-place-dvr #1("AlliGator Internal Variables DVR") -> (w24:T19, w20:errorcluster)
    n4 = in-place {
      in-place-border: w20 -> [w43]
      in-place-border: [w83] -> w22
      in-place-border: [w94] -> w21
      in-place-border: w19 -> [w91]
      n5 = in-place-cluster #2(w24) -> ("Fit Model"=w28:T10, "NLSF Parameters Map X Resolution"=w34:i32, "NLSF Parameters Map Y Resolution"=w33:i32, "Is Full Image Parameters Map"=w42:bool, "Current Dataset Images 1.SGL Image Sum"=w63:T4, "Current Dataset Images 1.SGL Gate Images"=w62:T4[], "Dual-Channel Dataset"=w58:bool, "Channel Arithmetic"=w57:T24, "Selected Channel Name"=w56:string, "Current Dataset Images 2.SGL Image Sum"=w61:T4, "Current Dataset Images 2.SGL Gate Images"=w60:T4[], "Reference Decay"=w49:cluster{"t Array":dbl[], "I Array":dbl[]}, "[[Multiple Decays Fit Parameters]]"=w76:dbl[][], "[Decay Fit Parameter Names]"=w73:T41[], "IRF Array Time Axis"=w71:dbl[], "[[IRFs]]"=w70:dbl[][], "Decay Fit Options & Parameters"=w67:T8, "Is Single-Pixels Parameters Map"=w29:bool, "[Decay Sum]"=w25:dbl[])
      n6 = call "AlliGator Get Pixel Count Constraints.vi"("error in (no error)"=w43) -> ("error out"=w101:errorcluster, "Pixel Count Constraints"=w102:T44)  [unwired: 9 in]
      n7 = call "AlliGator Settings Storage.vi"("AlliGator Settings List"=AlliGator_Settings_List."Fluorescence Decay_Decay Pre-Processing:Use Decay Pre-Processing", "Error In"=w43) -> ("Variant Data out"=w79:variant)  [unwired: 8 in, 1 out]
      n8 = call "Alligator Variables Storage.vi"("AlliGator Variable"=AlliGator_Variables_List."Files:Dataset Channel" ("Alligator Variable"), "Error In"=w43) -> ("Data out"=w45:variant)  [unwired: 7 in, 2 out]
      n9 = call "Alligator Variables Storage.vi"("AlliGator Variable"=AlliGator_Variables_List."Source Image:ROIs" ("Alligator Variable"), "Error In"=w43) -> ("Error Out"=w104:errorcluster, "Data out"=w105:variant)  [unwired: 7 in, 1 out]
      n10 = call-poly "Variant to Data.vi"("Variant"=w79) -> ("Value"=w77:bool)  [unwired: 8 in]
      n11 = call-poly "Variant to Data.vi"("Variant"=w45) -> ("U16 Value"=w44:u16)  [unwired: 8 in]
      n12 = call "AlliGator Settings Storage.vi"("AlliGator Settings List"=AlliGator_Settings_List."Fluorescence Decay_Advanced Analysis:Average Lifetime Options", "Error In"=w43) -> ("Error Out"=w55:errorcluster, "Variant Data out"=w52:variant)  [unwired: 8 in]
      n13 = call "AlliGator Settings Storage.vi"("AlliGator Settings List"=AlliGator_Settings_List."Fluorescence Decay_Fit Parameters:Export Tabulated Results", "Error In"=w43) -> ("Error Out"=w88:errorcluster, "Variant Data out"=w89:variant)  [unwired: 8 in]
      n14 = Variant To Data(error in=w104, type=T5[] [] ("Stored ROIs in"), Variant=w105) -> (data=w38:T5[], error out=w100:errorcluster)
      n15 = call-poly "Variant to Data.vi"("Variant"=w89) -> ("Value"=w81:bool)  [unwired: 8 in]
      n16 = Variant To Data(error in=w55, type=T2 {"Use Local IRF "=TRUE, "Use IRF Offset"=TRUE, "Use Fixed Offset"=TRUE, "Fixed Offset"=0.0, "Baseline %"=0.0} ("Average Lifetime Options"), Variant=w52) -> (data=w50:T2, error out=w53:errorcluster)
      n17 = Unbundle By Name(w50) -> ("Use Local IRF"=w48:bool)
      n18 = case shown="1" w44 {
        tunnel: [w108 w110] -> w64
        tunnel: w63 -> [w108 _]
        tunnel: [w107 w109] -> w65
        tunnel: w62 -> [w107 _]
        tunnel: w61 -> [_ w110]
        tunnel: w60 -> [_ w109]
        frame 0, Default {
        }
        frame 1 {
        }
      }
      n19 = Array Size(array=w38) -> (size(s)=w37:i32)
      n20 = Empty Array?(array=w38) -> (empty?=w47:bool)
      n21 = call "AlliGator Get Decay Peak Constraints.vi"("error in (no error)"=w43) -> ("Error Out"=w97:errorcluster, "Decay Peak Constraints"=w96:T47)  [unwired: 9 in]
      n22 = call "AlliGator Get Sum Image Threshold.vi"("error in (no error)"=w101, "Pixel Counts Constraints"=w102, "Image in"=w64) -> ("error out"=w93:errorcluster, "Pixel Threshold Low"=w98:sgl, "Pixel Threshold High"=w99:sgl, "Y Resolution"=w40:i32, "X Resolution"=w39:i32)  [unwired: 2 in, 2 out]
      n23 = Bundle By Name(cluster=cluster{"Image Sum":T4, "Image Array":T4[]} {"Image Sum"=refnum, "Image Array"=[]} ("Images"), "Image Sum"=w64, "Image Array"=w65) -> (w95:cluster{"Image Sum":T4, "Image Array":T4[]})
      n24 = Multiply(x=w39, y=w40) -> (x*y=w36:i32)
      n25 = Equal?(x=w37, y=w36) -> (x = y?=w35:bool)
      n26 = Merge Errors(w93, w100, w97, w53, w88) -> (w92:errorcluster)
      n27 = case shown="False" w47 {
        tunnel: w99 -> [w193 _]
        tunnel: w98 -> [w192 _]
        tunnel: w96 -> [w191 _]
        tunnel: w95 -> [w190 _]
        tunnel: w65 -> [w189 _]
        tunnel: w49 -> [w163 _]
        tunnel: [w123 _] -> w94
        tunnel: w92 -> [w172 _]
        tunnel: w91 -> [w148 _]
        tunnel: [w184 _] -> w87
        tunnel: [w114 _] -> w84
        tunnel: [w147 w315] -> w75
        tunnel: w81 -> [w183 _]
        tunnel: [w170 w316] -> w80
        tunnel: w38 -> [w182 _]
        tunnel: w77 -> [w181 _]
        tunnel: w76 -> [w169 w316]
        tunnel: w73 -> [w168 w314]
        tunnel: [w167 w314] -> w72
        tunnel: w71 -> [w166 w313]
        tunnel: w70 -> [w154 w312]
        tunnel: [w165 w313] -> w69
        tunnel: [w164 w312] -> w68
        tunnel: w67 -> [w160 w311]
        tunnel: [w159 w311] -> w66
        tunnel: w50 -> [w152 _]
        tunnel: w48 -> [w151 _]
        tunnel: w42 -> [w127 w310]
        tunnel: [w135 w310] -> w41
        tunnel: w35 -> [w128 _]
        tunnel: w34 -> [w132 w309]
        tunnel: w33 -> [w130 w308]
        tunnel: [w134 w309] -> w32
        tunnel: [w133 w308] -> w31
        tunnel: [w126 w307] -> w30
        tunnel: w29 -> [w125 w307]
        tunnel: w28 -> [w119 w306]
        tunnel: [w118 w306] -> w27
        tunnel: [w113 w305] -> w26
        tunnel: w25 -> [w112 w305]
        frame False {
          w155 = T41[] [enum."<tau>_i"] items=["Offset", "Baseline", "A_1", "tau_1", "A_2", "tau_2", "<tau>_a", "f1_a", "f2_a", "<tau>_i", "f1_i", "f2_i", "-", "R^2", "Chi^2"] ("f")
          n28 = Array Size(array=w189) -> (size(s)=w188:i32)
          n29 = call "Current Date & Time String (High Precision).vi"("Error In"=w172) -> ("Error Out"=w176:errorcluster, "on <Date> at <Time>"=w156:string)  [unwired: 7 in, 2 out]
          n30 = Unbundle By Name(w163) -> ("t Array"=w153:dbl[], "I Array"=w162:dbl[])
          n31 = Format Into String(format string="All ROIs Average Lifetimes Started %s", error in=w176, w156) -> (resulting string=w177:string, error out=w175:errorcluster)  [unwired: 1 in]
          n32 = call "AlliGator New NLSF Parameter Map Resolution.vi"("Is Full Image Parameter Map"=w128, "Old NLSF Parameters Map Y Resolution"=w130, "Old NLSF Parameters Map X Resolution"=w132) -> (2:"New NLSF Parameters Map X Resolution"=w129:i32, 3:"New NLSF Parameters Map X Resolution"=w131:i32)  [unwired: 7 in]
          n33 = Array Size(array=w182) -> (size(s)=w141:i32)
          n34 = call "Get Notebook Queue.vi"() -> ("Notebook Queue"=w174:refnum<queue>)  [unwired: 9 in]
          n35 = call "Get Current Message Text Format.vi"("Text Format"=Text_Format_List."Result") -> ("Message Formatting"=w179:T48)  [unwired: 8 in, 1 out]
          n36 = Build Array(w162) -> (w161:dbl[][])
          n37 = call "Send Message to Notebook.vi"("Text Formatting"=w179, "Error In"=w175, "Text"=w177, "Notebook Queue"=w174) -> ("Error Out"=w173:errorcluster)  [unwired: 4 in, 1 out]
          n38 = for {
            tunnel: w148 -> [w201]
            shift-right: [w203] -> w180
            shift-left: w173 -> [w199]
            tunnel: string[] ["<tau>", "<tau>_F", "t_0_F", "<tau>_IRF", " t_0_IRF"] ("initial string") -> [w194] mode=indexing
            n39 = Format Into String(format string=": %s", initial string="Multiple ROIs", error in=w199, w194) -> (resulting string=w197:string, error out=w198:errorcluster)
            n40 = call "XY Graph Try Plot Name.vi"("Error In"=w198, "Plot Name in"=w197, "XY Graph Refnum"=w201) -> ("Error Out"=w202:errorcluster, "Plot Name out"=w204:string, "XY Graph Refnum"=w195:T52)  [unwired: 5 in, 1 out]
            n41 = call "XY Graph Add New Plot.vi"("Multiplot XY Graph"=w195, "New Plot Name in"=w204, "error in (no error)"=w202) -> ("error out"=w203:errorcluster)  [unwired: 9 in, 3 out]
          }
          n42 = call "AlliGator Get Decay Time Axis v2.vi"("Number of Gates"=w188) -> ("t Array"=w187:dbl[unit][])  [unwired: 14 in]
          n43 = call "Embedded Progress Bar Q.vi"("Progress Bar Queue Name"="AlliGator Progress Bar Q") -> ("Progress Bar Queue"=w144:refnum<queue>)  [unwired: 6 in]
          n44 = call "AlliGator Get-Set Decay Preprocessing Parameters.vi"("Get (F)/Set"=FALSE, "Error In"=w180) -> ("Error Out"=w145:errorcluster, "Decay Preprocessing Parameters out"=w158:T40)  [unwired: 8 in]
          n45 = node(w187) -> (w186:dbl[])
          n46 = call "Logical Processors Used.vi"() -> ()  [unwired: 6 in, 1 out]
          n47 = call "Send Embedded Progress Bar Update.vi"("Max Iterations N"=w141, "Current Iteration i (i or -1: standard or || iteration; 0 or -2: first standard or || iteration)"=-2 ("Current Iteration i (i or -1: standard or || iteration; 0 or -2: first standard or || iteration)"), "Progress Bar Queue in"=w144) -> ("Error Out"=w139:errorcluster, "Progress Bar Queue out"=w140:refnum<queue>)  [unwired: 7 in]
          n48 = for {
            tunnel: w182 -> [w238] mode=indexing
            tunnel: w193 -> [w237]
            tunnel: w192 -> [w236]
            tunnel: w190 -> [w235]
            tunnel: w191 -> [w234]
            tunnel: w186 -> [w232]
            tunnel: w163 -> [w218]
            tunnel: [w231] -> w123 mode=indexing if=w224
            tunnel: w145 -> [w233]
            tunnel: [FALSE ("Abort?")] -> w185
            tunnel: "Abort Fit" ("Abort Button Name (Abort)") -> [w229]
            tunnel: [w228] -> w184 mode=indexing if=w205
            tunnel: w183 -> [w227]
            tunnel: [w214] -> w114
            tunnel: [w215] -> w171 mode=indexing if=w205
            tunnel: w141 -> [w226]
            tunnel: w181 -> [w222]
            tunnel: w158 -> [w221]
            tunnel: w154 -> [w220]
            tunnel: w153 -> [w219]
            tunnel: w152 -> [w216]
            tunnel: w151 -> [w217]
            tunnel: [w213] -> w149 mode=indexing if=w205
            tunnel: w140 -> [w211]
            tunnel: w139 -> [w210]
            tunnel: [w209] -> w137
            tunnel: [w208] -> w136
            tunnel: [w207] -> w124 mode=indexing if=w205
            tunnel: [w206] -> w115 mode=indexing if=w205
            i -> [w225]
            n49 = global read "AlliGator Abort.vi" "Abort?"() -> (w214:bool)
            n50 = case shown="False" w214 {
              tunnel: w238 -> [w280 _]
              tunnel: w237 -> [w279 _]
              tunnel: w236 -> [w278 _]
              tunnel: w235 -> [w277 _]
              tunnel: w234 -> [w276 _]
              tunnel: w233 -> [w275 _]
              tunnel: w232 -> [w272 _]
              tunnel: [w268 _] -> w231
              tunnel: w229 -> [_ _]
              tunnel: [w267 _] -> w228
              tunnel: w227 -> [w266 _]
              tunnel: w226 -> [w265 _]
              tunnel: w225 -> [w242 _]
              tunnel: [w264 _] -> w223
              tunnel: [w263 _] -> w205
              tunnel: w222 -> [w260 _]
              tunnel: w221 -> [w259 _]
              tunnel: w220 -> [w257 _]
              tunnel: w219 -> [w256 _]
              tunnel: w218 -> [w255 _]
              tunnel: w217 -> [w250 _]
              tunnel: w216 -> [w249 _]
              tunnel: [w246 _] -> w215
              tunnel: [w245 _] -> w213
              tunnel: [w243 _] -> w207
              tunnel: [w239 _] -> w206
              frame False {
                n51 = Unbundle By Name(w280) -> ("ROI Descriptor"=w274:T6, "ROI Name"=w268:string)
                n52 = call "AlliGator Compute ROI Decay.vi"("Pixel Threshold High"=w279, "Loop ID"=w242, "Pixel Threshold Low"=w278, "error in (no error)"=w275, "Decay Peak  Constraints"=w276, "ROI Descriptor"=w274, "Images"=w277) -> ("error out"=w273:errorcluster, "# Valid Pixels"=w269:i32, "ROI Center"=w258:cluster{"X":i32, "Y":i32}, "Decay Points"=w271:dbl[], "# Pixels"=w243:i32)
                n53 = Cluster To Array(cluster=w258) -> (array=w262:i32[])
                n54 = Bundle(w272, "Decay Points"=w271) -> (w270:cluster{dbl[], "Decay Points":dbl[]})  [unwired: 1 in]
                n55 = To Double Precision Float(number=w262) -> (double precision float=w261:dbl[])
                n56 = case shown="True" w260 {
                  tunnel: w273 -> [w293 w301]
                  tunnel: w270 -> [w294 w300]
                  tunnel: w269 -> [_ w299]
                  tunnel: [w293 w298] -> w244
                  tunnel: w255 -> [_ w297]
                  tunnel: [w294 w296] -> w241
                  tunnel: w259 -> [_ w295]
                  frame False {
                  }
                  frame True {
                    n57 = call "AlliGator Preprocess Decay v3.vi"("Decay Preprocessing Parameters"=w295, "Error In"=w301, "Time-Gated Reference Decay"=w297, "# Pixels"=w299, "Decay (in)"=w300) -> ("Error Out"=w298:errorcluster, "Decay (out)"=w296:T53)  [unwired: 3 in, 2 out]
                  }
                }
                n58 = call "Keep String in Array.vi"("Current Index"=w242, "Number of Elements"=w265) -> ("Keep String"=w264:bool)  [unwired: 9 in]
                n59 = case shown="True" w250 {
                  tunnel: w257 -> [_ w292]
                  tunnel: w255 -> [w281 w289]
                  tunnel: [w281 w288] -> w254
                  tunnel: w256 -> [_ w287]
                  tunnel: w258 -> [_ w284]
                  frame False {
                  }
                  frame True {
                    # "Look for local IRF"
                    n60 = call "AlliGator Get IRF Values & Locations.vi"("[IRF Data]"=w292) -> ("IRF Locations"=w282:cluster{"X":i32, "Y":i32}[], "[IRF Values]"=w283:dbl[][])  [unwired: 9 in]
                    n61 = Search 1D Array(1D array=w282, element=w284) -> (index of element=w291:i32)  [unwired: 1 in]
                    n62 = Index Array(array=w283, index (row)=w291) -> (element=w286:dbl[])  [unwired: 1 in]
                    n63 = Less Than 0?(x=w291) -> (x < 0?=w290:bool)
                    n64 = Bundle("t Array"=w287, "[IRF Values]"=w286) -> (w285:cluster{"t Array":dbl[], "[IRF Values]":dbl[]})  [unwired: 1 in]
                    n65 = Select(t=w289, s=w290, f=w285) -> (s? t:f=w288:cluster{"t Array":dbl[], "[IRF Values]":dbl[]})
                  }
                }
                n66 = call "AlliGator Computer IRF t_0 and Mean Lifetime.vi"("error in"=w244, "Reference Decay"=w254) -> ("error out"=w251:errorcluster, "t_0"=w252:dbl, "<tau>_IRF"=w253:dbl)  [unwired: 7 in]
                n67 = Unbundle By Name(w241) -> ("ROI Intensity Array"=w240:dbl[])
                n68 = call "AlliGator Compute Decay Average Lifetime.vi"("Average Lifetime Options"=w249, "error in (no error)"=w251, "t_0_IRF"=w252, "<tau>_IRF"=w253, "Plot"=w241) -> ("error out"=w248:errorcluster, "Average Lifetime Outputs"=w245:dbl[])  [unwired: 5 in]
                n69 = Unbundle By Name(w248) -> ("status"=w247:bool)
                n70 = Add Array Elements(numeric array=w240) -> (sum=w239:dbl)
                n71 = Build Array (concatenate)(w261, w245) -> (w246:dbl[])
                n72 = Not(x=w247) -> (.not. x?=w263:bool)
                n73 = case shown="True" w266 {
                  tunnel: [_ w304] -> w267
                  tunnel: w246 -> [_ w303]
                  frame False {
                  }
                  frame True {
                    n74 = Array To Spreadsheet String(array=w303, 3:"%#g" ("format string")) -> (spreadsheet string=w304:string)  [unwired: 1 in]
                  }
                }
              }
              frame True {
              }
            }
            n75 = call "Send Embedded Progress Bar Update.vi"("Error In"=w210, "Current Iteration i (i or -1: standard or || iteration; 0 or -2: first standard or || iteration)"=-1 ("Current Iteration i (-1: || iteration, -2: first || iteration)"), "Progress Bar Queue in"=w211) -> ("Error Out"=w208:errorcluster, "Progress Bar Queue out"=w209:refnum<queue>)  [unwired: 7 in]
            n76 = Compound Arithmetic op=AND(w223, w205) -> (w224:bool)
          }
          n77 = global write "AlliGator Abort.vi" "Abort?"(w185) -> ()
          n78 = Add Array Elements(numeric array=w124) -> (sum=w121:i32)
          n79 = call "Send Embedded Progress Bar Update.vi"("Stop Progress Bar (F)"=TRUE, "Error In"=w136, "Progress Bar Queue in"=w137) -> ()  [unwired: 7 in, 2 out]
          n80 = Select(t=w130, s=w114, f=w129) -> (s? t:f=w133:i32)
          n81 = Select(t=w169, s=w114, f=w171) -> (s? t:f=w170:dbl[][])
          n82 = Array Size(array=w123) -> (size(s)=w122:i32)
          n83 = Select(t=w168, s=w114, f=w155) -> (s? t:f=w167:T41[])
          n84 = Select(t=w132, s=w114, f=w131) -> (s? t:f=w134:i32)
          n85 = call "XY Graph Add Data to Last Plots.vi"("Plots Data Array"=w149, "XYGraph in"=w148) -> ("error out"=w147:errorcluster)  [unwired: 9 in]
          n86 = Select(t=w154, s=w114, f=w161) -> (s? t:f=w164:dbl[][])
          n87 = Select(t=w166, s=w114, f=w153) -> (s? t:f=w165:dbl[])
          n88 = Select(t=w160, s=w114, f=T8 {"SYNC Period"=0.0, "Fit Options"={"Show Fit Residuals"=FALSE, "Fit Model"=enum."1-Exponential", "Residual Type"=enum."Standard", "Max Decay Percentile"=0.0, "Min Decay Percentile"=0.0, "Show Full Decay"=FALSE, "Weights"=enum."Unweighted", "Fitting Method"=enum."Least Square", "Compute Parameter Uncertainties"=FALSE, "Periodic Boundaries"=FALSE, "Model Calculation"=enum."Simulation", "Period"=0.0, "Termination Criteria"={"Max Iterations"=0, "Max Function Calls"=0, "Max Time"=0.0, "Function Tolerance"=0.0, "Parameter Tolerance"=0.0, "Gradient Tolerance"=0.0, "Min Lambda"=0.0, "Max Lambda"=0.0, "Initial Tick Count"=0}, "Offset Resolution"=0.0, "Use Local IRF"=FALSE, "Fitting Algorithm"=enum."Levenberg-Marquardt", "Show Confidence Interval "=TRUE, "Confidence Level"=95.0}, "Fit Parameter Constraints"=[], "MLE Baseline Offset"=0.0, "MLE Baseline Offset Type"=enum."Absolute"}) -> (s? t:f=w159:T8)
          n89 = Select(t=w127, s=w114, f=w128) -> (s? t:f=w135:bool)
          n90 = Equal?(x=w122, y=w121) -> (x = y?=w120:bool)
          n91 = Select(t=w119, s=w114, f=Decay_Model."1-Exponential") -> (s? t:f=w118:T10)
          n92 = Select(t=w125, s=w114, f=w120) -> (s? t:f=w126:bool)
          n93 = Select(t=w115, s=w114, f=w112) -> (s? t:f=w113:dbl[])
        }
        frame True {
          n94 = xnode "Error Ring"() -> ("error out"=w315:errorcluster)
        }
      }
      n95 = in-place-cluster #2("Fit Model"=w27, "NLSF Parameters Map X Resolution"=w32, "NLSF Parameters Map Y Resolution"=w31, "Is Full Image Parameters Map"=w41, "Current Dataset Images 1.SGL Image Sum"=w63, "Current Dataset Images 1.SGL Gate Images"=w62, "Dual-Channel Dataset"=w58, "Channel Arithmetic"=w57, "Selected Channel Name"=w56, "Current Dataset Images 2.SGL Image Sum"=w61, "Current Dataset Images 2.SGL Gate Images"=w60, "Reference Decay"=w49, "[[Multiple Decays Fit Parameters]]"=w80, "[Decay Fit Parameter Names]"=w72, "IRF Array Time Axis"=w69, "[[IRFs]]"=w68, "Decay Fit Options & Parameters"=w66, "Is Single-Pixels Parameters Map"=w30, "[Decay Sum]"=w26) -> (w23:T19)
      n96 = call "AlliGator Get Tabulated Results Header (Average Lifetimes).vi"("Error In"=w75) -> ("Error Out"=w74:errorcluster, "Tabulated Results Header"=w86:string)  [unwired: 9 in]
      n97 = Build Array (concatenate)(w86, w87) -> (w85:string[])
      n98 = case shown="False" w84 {
        tunnel: w85 -> [w325 _]
        tunnel: [w324 w331] -> w83
        tunnel: w74 -> [w323 w331]
        tunnel: "Choose or enter file path for tabulated average lifetimea results:" ("prompt (Choose or enter file path)") -> [w322 _]
        tunnel: w81 -> [w321 _]
        frame False {
          n99 = case shown="True" w321 {
            tunnel: w325 -> [_ w330]
            tunnel: [w326 w329] -> w324
            tunnel: w323 -> [w326 w328]
            tunnel: w322 -> [_ w327]
            frame False {
            }
            frame True {
              n100 = Write to Text File(prompt (Choose or enter file path)=w327, text=w330, error in=w328) -> (error out=w329:errorcluster)  [unwired: 1 in, 2 out]
            }
          }
        }
        frame True {
        }
      }
    }
    n101 = in-place-dvr #1(w23) -> (→"AlliGator Internal Variables DVR":refnum<data-value>)  [unwired: 1 out]
  }
  n102 = call "High Resolution Timing.vi"("relative seconds (NaN)"=w12, "Error In"=w5) -> ("elapsed (relative) seconds"=w11:dbl, "Error Out"=w6:errorcluster)  [unwired: 15 in, 1 out]
  n103 = Array Size(array=w9) -> (size(s)=w8:i32)
  n104 = call "Concatenate String Array.vi"("Max Number of Elements (None: -1)"=8 ("Max Number of Elements (None: 1)"), "Separator (TAB)"=", ", "String Array"=w9) -> ("Formatted String"=w10:string)  [unwired: 8 in]
  n105 = call "Current Date & Time String (High Precision).vi"("Error In"=w6) -> ("on <Date> at <Time>"=w1:string)  [unwired: 7 in, 3 out]
  n106 = Format Into String(format string="All ROIs Average Lifetimes (%d):\n%scompleted %s\nCPU: %#g s\n", error in=w6, w8, w10, w1, w11) -> (resulting string=→"Message":string, error out=→"error out":errorcluster)  [unwired: 1 in]
